vi "Make VI Param(Read Batch Profile Storage Rsp).vi"(1 "pRsp":T3) -> (0 "Read Batch Profile Storage Rsp":T1)   [LabVIEW 8.6, in "Keyence LJ-V7000.lvlib"]
uses:
  Keyence LJ-V7000.lvlib
  Public/Clusters/Time.ctl
  Public/Clusters/Read Batch Profile Storage Rsp.ctl
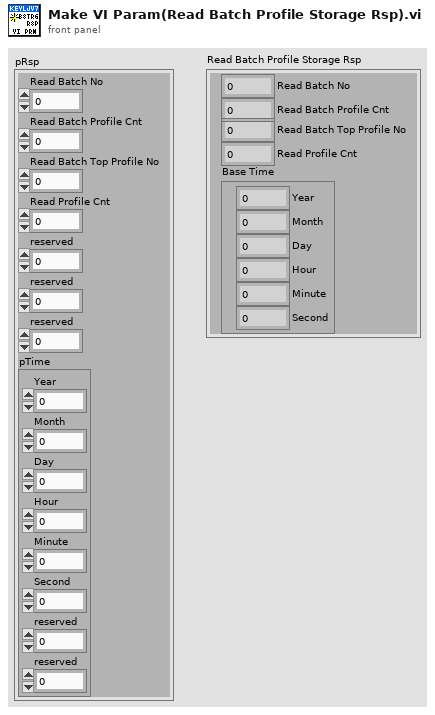
[diagram p1: front panel]
types:
  T1 = typedef "Keyence LJ-V7000.lvlib/Read Batch Profile Storage Rsp.ctl" = cluster{"Read Batch No":u32, "Read Batch Profile Cnt":u32, "Read Batch Top Profile No":u32, "Read Profile Cnt":u8, "Base Time":T2}
  T2 = typedef "Keyence LJ-V7000.lvlib/Time.ctl" = cluster{"Year":u8, "Month":u8, "Day":u8, "Hour":u8, "Minute":u8, "Second":u8}
  T3 = cluster{"Read Batch No":u32, "Read Batch Profile Cnt":u32, "Read Batch Top Profile No":u32, "Read Profile Cnt":u8, "reserved":u8, "reserved":u8, "reserved":u8, "pTime":cluster{"Year":u8, "Month":u8, "Day":u8, "Hour":u8, "Minute":u8, "Second":u8, "reserved":u8, "reserved":u8}}
  T4 = cluster{"Year":u8, "Month":u8, "Day":u8, "Hour":u8, "Minute":u8, "Second":u8, "reserved":u8, "reserved":u8}
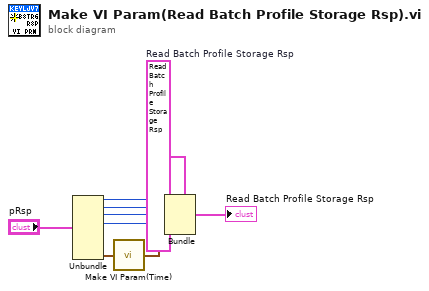
[diagram p0: block diagram]
diagram:
  w2 = T1 ?  # Read Batch Profile Storage Rsp
  n1 = Unbundle("pRsp") -> ("Read Batch No"=w8:u32, "Read Batch Profile Cnt"=w7:u32, "Read Batch Top Profile No"=w6:u32, "Read Profile Cnt"=w5:u8, "pTime"=w4:T4)  [unwired: 3 out]
  n2 = call "Make VI Param(Time).vi"("pTime"=w4) -> ("Time"=w3:T2)
  n3 = Bundle(cluster=w2, "Read Batch No"=w8, "Read Batch Profile Cnt"=w7, "Read Batch Top Profile No"=w6, "Read Profile Cnt"=w5, "Base Time"=w3) -> (→"Read Batch Profile Storage Rsp":T1)
